vi "tragetory generation.vi"(11 "file path":path) -> (3 "reference":dbl)   [LabVIEW 2018, in "kevLib2010.lvlib"]
uses:
  kevLib2010.lvlib
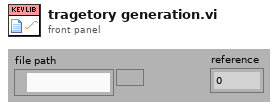
[diagram p1: front panel]
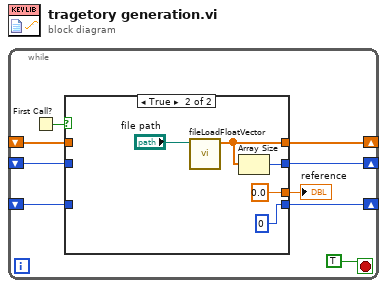
[diagram p0: block diagram]
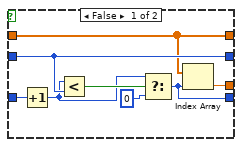
[diagram p2: hidden frame]
diagram:
  n1 = while {
    shift-right: [w6] -> _
    shift-left: _ -> [w4]
    shift-right: [w7] -> _
    shift-left: _ -> [w5]
    shift-right: [w3] -> _
    shift-left: _ -> [w2]
    stop <- TRUE stop-if-true
    n2 = First Call?() -> (First Call?: T/F=w9:bool)
    n3 = case shown="True" w9 {
      tunnel: [w16 w19] -> w7
      tunnel: [w13 w18] -> w6
      tunnel: w5 -> [w16 _]
      tunnel: w4 -> [w13 _]
      tunnel: [w12 0 ("f")] -> w3
      tunnel: w2 -> [w15 _]
      tunnel: [w11 0.0 ("Data Type (DBL)")] -> w1
      frame False {
        n4 = Increment(x=w15) -> (x+1=w10:i32)
        n5 = Less?(x=w10, y=w16) -> (x < y?=w17:bool)
        n6 = Select(t=w10, s=w17, f=0) -> (s? t:f=w12:i32)
        n7 = Index Array(array=w13, index=w12) -> (element=w11:dbl)
      }
      frame True {
        n8 = call "fileLoadFloatVector.vi"("File Path"="file path") -> ("Float Vector"=w18:dbl[])  [unwired: 9 in, 1 out]
        n9 = Array Size(array=w18) -> (size(s)=w19:i32)
      }
    }
    "reference" <- w1
  }
